vi "Serialize as XML.vi"(8 "error in (no error)":errorcluster, 11 "Element in":refnum<class "Element.lvclass">) -> (0 "error out":errorcluster, 2 "XML Fragment":string, 3 "Element out":refnum<class "Element.lvclass">)   [LabVIEW 2023, in "VILab.lvlib" / "Element.lvclass"]
uses:
  Element.lvclass
  Element.lvclass/Element.ctl
  Attribute/Attribute.lvclass
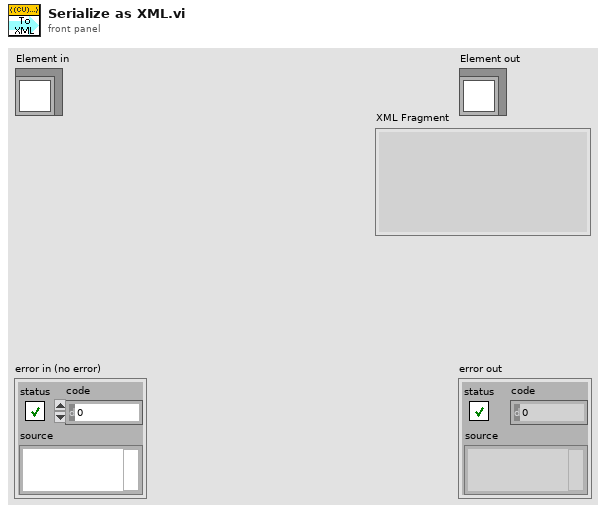
[diagram p1: front panel]
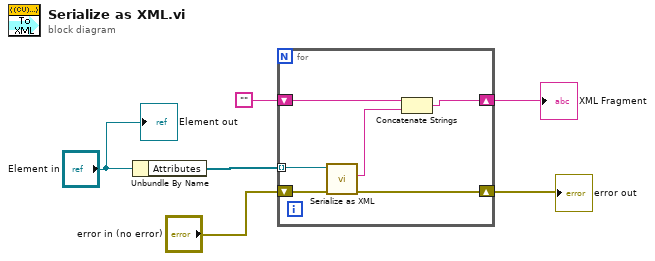
[diagram p0: block diagram]
diagram:
  n1 = Unbundle By Name("Element in") -> ("Attributes"=w5:refnum<class "Attribute.lvclass">[])
  n2 = for {
    tunnel: w5 -> [w11] mode=indexing
    shift-right: [w8] -> w1
    shift-left: "" -> [w12]
    shift-right: [w7] -> w2
    shift-left: "error in (no error)" -> [w10]
    n3 = call-dynamic "Serialize as XML.vi"("error in (no error)"=w10, "Attribute in"=w11) -> ("error out"=w7:errorcluster, "XML Fragment"=w9:string)  [unwired: 7 in, 1 out]
    n4 = Concatenate Strings(w12, w9) -> (w8:string)
  }
  "error out" <- w2
  "XML Fragment" <- w1
  "Element out" <- "Element in"
